vi "Global.vi"() -> ()   [LabVIEW 2013]
panel:
  in  "DisengagedAngle":dbl
  in  "EngagedAngle":dbl
  in  "Launch?":bool
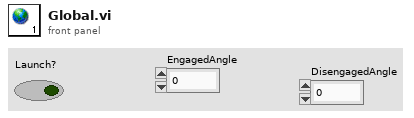
[diagram p1: front panel]
diagram:
